vi "GetSubset.vi"(8 "SubCut":cluster{dbl, dbl}={0.0, 1.0}, 10 "Commands in":string[](array[string]), 11 "cmd amd State":cluster{"Command":string, "End State":dbl[]}[](array[cluster])) -> (2 "Commands out":string[](array[string]), 3 "cmd amd State out":cluster{"Command":string, "End State":dbl[]}[](array[cluster]))   [LabVIEW 2024]
panel:
  out "Header Length":i32
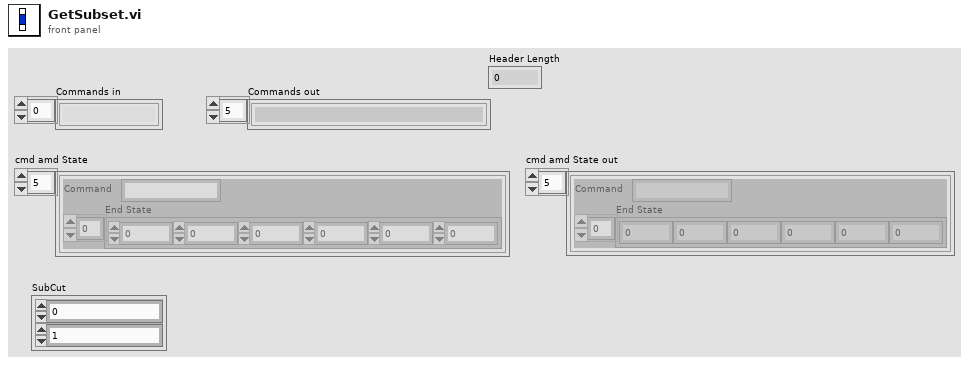
[diagram p1: front panel]
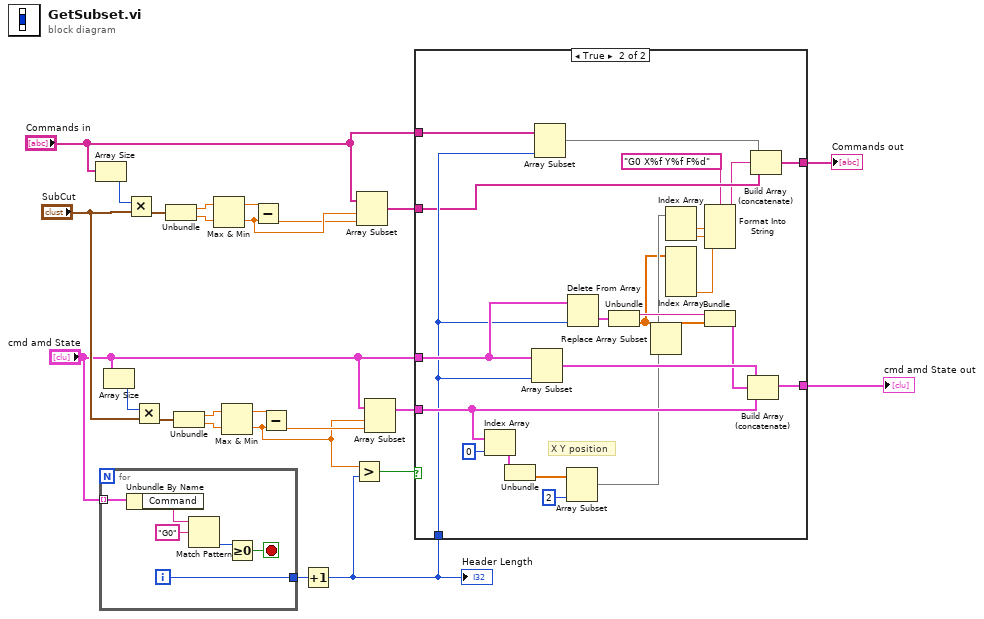
[diagram p0: block diagram]
diagram:
  n1 = Array Size(array="Commands in") -> (size(s)=w22:i32)
  n2 = for {
    tunnel: "cmd amd State" -> [w30] mode=indexing
    tunnel: [w25] -> w6
    i -> [w25]
    stop <- w26 stop-if-true
    n3 = Unbundle By Name(w30) -> ("Command"=w29:string)
    n4 = Match Pattern(string=w29, regular expression="G0") -> (offset past match=w27:i32)  [unwired: 1 in, 3 out]
    n5 = Greater Or Equal To 0?(x=w27) -> (x >= 0?=w26:bool)
  }
  n6 = Array Size(array="cmd amd State") -> (size(s)=w14:i32)
  n7 = Multiply(x=w22, y="SubCut") -> (x*y=w21:cluster{dbl, dbl})
  n8 = Multiply(x=w14, y="SubCut") -> (x*y=w15:cluster{dbl, dbl})
  n9 = Unbundle(w21) -> (w24:dbl, w23:dbl)
  n10 = Unbundle(w15) -> (w12:dbl, w13:dbl)
  n11 = Max & Min(x=w24, y=w23) -> (max(x,y)=w20:dbl, min(x,y)=w19:dbl)
  n12 = Max & Min(x=w12, y=w13) -> (max(x,y)=w16:dbl, min(x,y)=w7:dbl)
  n13 = Subtract(x=w20, y=w19) -> (x-y=w18:dbl)
  n14 = Subtract(x=w16, y=w7) -> (x-y=w17:dbl)
  n15 = Increment(x=w6) -> (x+1=w4:i32)
  "Header Length" <- w4
  n16 = Greater?(x=w7, y=w4) -> (0:w5:bool)
  n17 = Array Subset(array="Commands in", index=w19, length=w18) -> (w2:string[])
  n18 = Array Subset(array="cmd amd State", index=w7, length=w17) -> (w9:cluster{"Command":string, "End State":dbl[]}[])
  n19 = case shown="True" w5 {
    tunnel: "cmd amd State" -> [w32 w49]
    tunnel: w9 -> [_ w48]
    tunnel: [w32 w56] -> w8
    tunnel: w4 -> [_ w42]
    tunnel: "Commands in" -> [w31 w43]
    tunnel: w2 -> [_ w41]
    tunnel: [w31 w40] -> w1
    frame False {
    }
    frame True {
      # "X Y position"
      n20 = Index Array(array=w48, index=0) -> (element=w55:cluster{"Command":string, "End State":dbl[]})
      n21 = Unbundle(w55) -> ("End State"=w46:dbl[])  [unwired: 1 out]
      n22 = Array Subset(array=w49, length=w42) -> (w54:cluster{"Command":string, "End State":dbl[]}[])  [unwired: 1 in]
      n23 = Array Subset(array=w43, length=w42) -> (w44:string[])  [unwired: 1 in]
      n24 = Array Subset(array=w46, length=2 ("index")) -> (w38:dbl[])  [unwired: 1 in]
      n25 = Delete From Array(array=w49, index=w42) -> (deleted portion=w53:cluster{"Command":string, "End State":dbl[]})  [unwired: 1 in, 1 out]
      n26 = Unbundle(w53) -> ("Command"=w52:string, "End State"=w35:dbl[])
      n27 = Replace Array Subset(array=w35, new element=w38) -> (w51:dbl[])  [unwired: 1 in]
      n28 = Index Array(array=w38) -> (element #1=w37:dbl, element #2=w36:dbl)  [unwired: 2 in]
      n29 = Index Array(array=w35) -> (element #4=w34:dbl)  [unwired: 4 in, 3 out]
      n30 = Format Into String(format string="G0 X%f Y%f F%d" ("regular expression"), w37, w36, w34) -> (resulting string=w33:string)  [unwired: 2 in, 1 out]
      n31 = Bundle("Command"=w52, "End State"=w51) -> (w50:cluster{"Command":string, "End State":dbl[]})  [unwired: 1 in]
      n32 = Build Array (concatenate)(w54, w50, w48) -> (w56:cluster{"Command":string, "End State":dbl[]}[])
      n33 = Build Array (concatenate)(w44, w33, w41) -> (w40:string[])
    }
  }
  "Commands out" <- w1
  "cmd amd State out" <- w8
